vi "Scripting_IndicateConnectorPaneCorners.vi"(10 "Terminals[]":refnum<vi>[](array[refnum]), 11 "TermBnds[]":T1[](array[typedef])) -> (0 "RightLower":i32, 1 "LeftLower":i32, 2 "RightTop":i32, 3 "LeftTop":i32)   [LabVIEW 2014]
uses:
  <vilib>/Utility/miscctls.llb/LVRectTypeDef.ctl
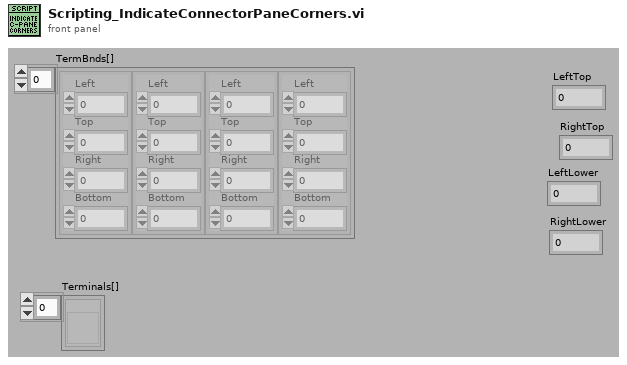
[diagram p1: front panel]
types:
  T1 = typedef "LVRectTypeDef.ctl" = cluster{"Left":i16, "Top":i16, "Right":i16, "Bottom":i16}
  T2 = typedef "LVPositionTypeDef.ctl" = cluster{"Left":i32, "Top":i32}
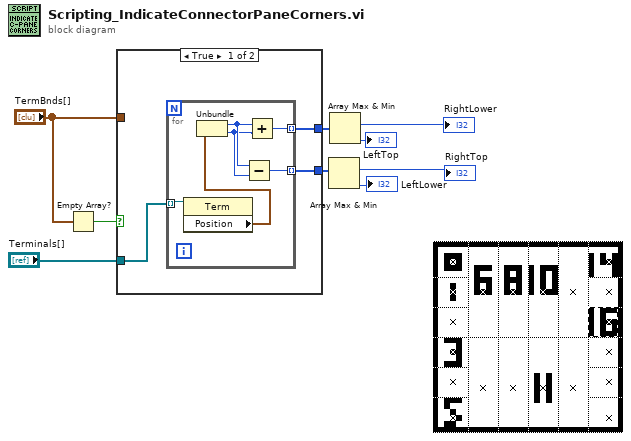
[diagram p0: block diagram]
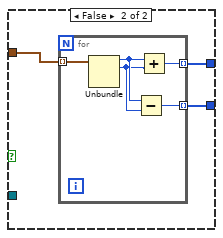
[diagram p2: hidden frame]
diagram:
  n1 = Empty Array?(array="TermBnds[]") -> (empty?=w2:bool)
  n2 = case shown="True" w2 {
    tunnel: [w12 w21] -> w9
    tunnel: [w11 w20] -> w8
    tunnel: "TermBnds[]" -> [_ w19]
    tunnel: "Terminals[]" -> [w10 _]
    frame True {
      n3 = for {
        tunnel: [w18] -> w12 mode=indexing
        tunnel: [w17] -> w11 mode=indexing
        tunnel: w10 -> [w14] mode=indexing
        n4 = property class="Term"(reference=w14) -> ("Position"=w13:T2)  [unwired: 1 in, 2 out]
        n5 = Unbundle(w13) -> ("Left"=w16:i32, "Top"=w15:i32)
        n6 = Subtract(x=w16, y=w15) -> (x-y=w17:i32)
        n7 = Add(x=w16, y=w15) -> (x+y=w18:i32)
      }
    }
    frame False {
      n8 = for {
        tunnel: w19 -> [w26] mode=indexing
        tunnel: [w25] -> w21 mode=indexing
        tunnel: [w24] -> w20 mode=indexing
        n9 = Unbundle(w26) -> ("Left"=w23:i16, "Top"=w22:i16)  [unwired: 2 out]
        n10 = Subtract(x=w23, y=w22) -> (x-y=w24:i16)
        n11 = Add(x=w23, y=w22) -> (x+y=w25:i16)
      }
    }
  }
  n12 = Array Max & Min(array=w8) -> (max index (indices)=→"RightTop":i32, min index (indices)=→"LeftLower":i32)  [unwired: 2 out]
  n13 = Array Max & Min(array=w9) -> (max index (indices)=→"RightLower":i32, min index (indices)=→"LeftTop":i32)  [unwired: 2 out]
